vi "find facing.vi"(10 "Robot Angle":dbl, 11 "TeleOp Data Cluster":T1) -> (3 "Facing":dbl)   [LabVIEW 2018]
uses:
  TypeDefs/Teleop Data Cluster.ctl
panel:
  in  "GYRO":dbl format="%#_13g"
  in  "POV":i32
  out "compass":dbl
  out "Left?":bool
  out "Adjusted Compass":dbl
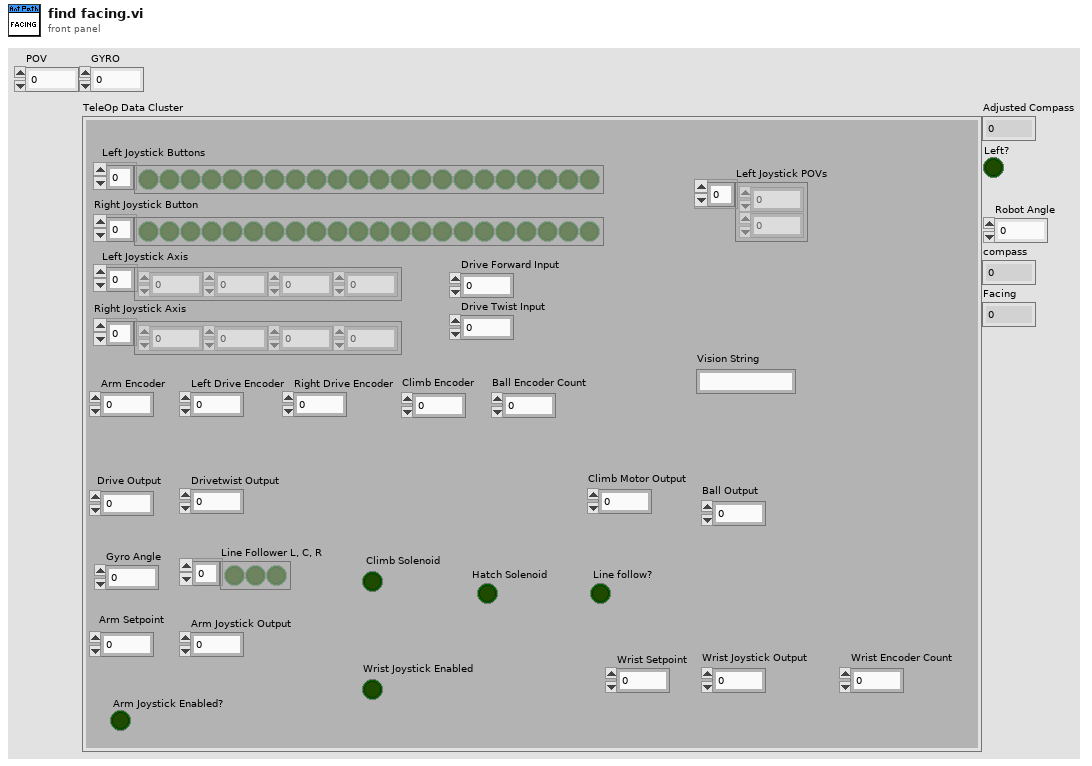
[diagram p1: front panel]
types:
  T1 = typedef "Teleop Data Cluster.ctl" = cluster{"Drive Forward Input ":dbl, "Drive Twist Input":dbl, "Drive Output":dbl, "Drivetwist Output":dbl, "Left Joystick Buttons":bool[], "Left Joystick Axis":dbl[], "Right Joystick Axis":dbl[], "Right Joystick Button":bool[], "Arm Encoder":dbl, "Left Drive Encoder":dbl, "Right Drive Encoder":dbl, "Gyro Angle ":dbl, "Arm Joystick Output  ":dbl, "Line Follower L, C, R ":bool[], "Line follow?":bool, " Climb Solenoid":bool, "Wrist Encoder Count":dbl, "Wrist Joystick Output":dbl, "Ball Encoder Count":dbl, "Ball Output":dbl, "Climb Encoder":dbl, "Climb Motor Output":dbl, " Hatch Solenoid":bool, "Arm Setpoint ":dbl, "Wrist Setpoint ":dbl, "Arm Joystick Enabled?":bool, "Wrist Joystick Enabled":bool, "Vision String":string, "Left Joystick POVs":i16[]}
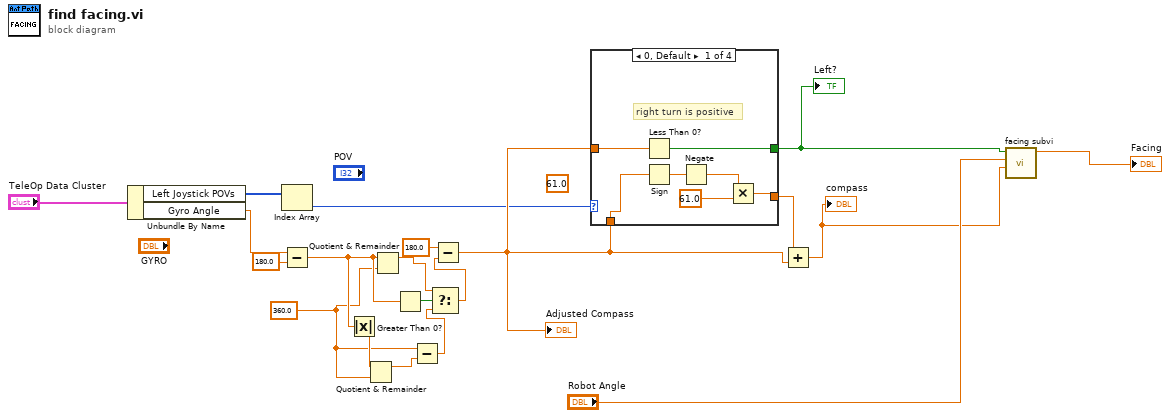
[diagram p0: block diagram]
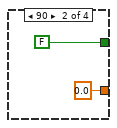
[diagram p2: hidden frame]
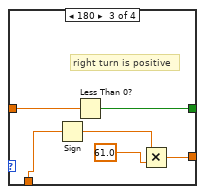
[diagram p3: hidden frame]
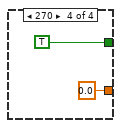
[diagram p4: hidden frame]
diagram:
  (unwired) 61.0
  w2 = 360.0 ("y")
  n1 = Unbundle By Name("TeleOp Data Cluster") -> ("Left Joystick POVs"=w19:i16[], "Gyro Angle"=w1:dbl)
  n2 = Index Array(array=w19) -> (element=w10:i16)  [unwired: 1 in]
  n3 = Subtract(x=w1, y=180.0) -> (x-y=w8:dbl)
  n4 = Absolute Value(x=w8) -> (abs(x)=w9:dbl)
  n5 = Quotient & Remainder(x=w9, y=w2) -> (x-y*floor(x/y)=w4:dbl)  [unwired: 1 out]
  n6 = Quotient & Remainder(x=w8, y=w2) -> (x-y*floor(x/y)=w6:dbl)  [unwired: 1 out]
  n7 = Greater Than 0?(x=w8) -> (x > 0?=w7:bool)
  n8 = Subtract(x=w2, y=w4) -> (x-y=w3:dbl)
  n9 = Select(t=w6, s=w7, f=w3) -> (s? t:f=w5:dbl)
  n10 = Subtract(x=180.0, y=w5) -> (x-y=w15:dbl)
  "Adjusted Compass" <- w15
  n11 = case shown="0, Default" w10 {
    tunnel: w15 -> [w27 _ w35 _]
    tunnel: [w26 FALSE w34 TRUE] -> w14
    tunnel: [w23 0.0 w31 0.0] -> w16
    tunnel: w15 -> [w22 _ w30 _]
    frame 0, Default {
      # "right turn is positive"
      n12 = Less Than 0?(x=w27) -> (x < 0?=w26:bool)
      n13 = Sign(1:w22) -> (0:w25:dbl)
      n14 = Negate(x=w25) -> (-x=w21:dbl)
      n15 = Multiply(x=w21, y=61.0) -> (x*y=w23:dbl)
    }
    frame 90 {
    }
    frame 180 {
      # "right turn is positive"
      n16 = Sign(1:w30) -> (0:w32:dbl)
      n17 = Less Than 0?(x=w35) -> (x < 0?=w34:bool)
      n18 = Multiply(x=w32, y=61.0) -> (x*y=w31:dbl)
    }
    frame 270 {
    }
  }
  "Left?" <- w14
  n19 = Add(x=w16, y=w15) -> (x+y=w12:dbl)
  "compass" <- w12
  n20 = call "facing subvi.vi"("Compass"=w12, "Robot Angle"="Robot Angle", "Left?"=w14) -> ("Facing"=→"Facing":dbl)  [unwired: 8 in]
